vi "Shallow Copy.vi"(7 "Tree ID":string, 8 "Error In":errorcluster, 11 "Tree Manager":T1) -> (0 "Error Out":errorcluster, 3 "Tree Manager":T1, 5 "Unique ID of Copied Tree":string)   [LabVIEW 2016, in "Tree Manager.lvclass"]
doc: "Shallow copy of a Tree and its attributes. Does not copy the Children of the Tree. On all attributes that are Tree Data types a Copy method is invoked. Overwrite the Copy the method in child types of Tree Data to implement special copying mechanism. The Default mechanism is copying by values i.e. LV fork."
uses:
  Tree Manager.lvclass
  Typedefs/Session Handle.ctl
  Tree Manager.lvclass/Tree Manager.ctl
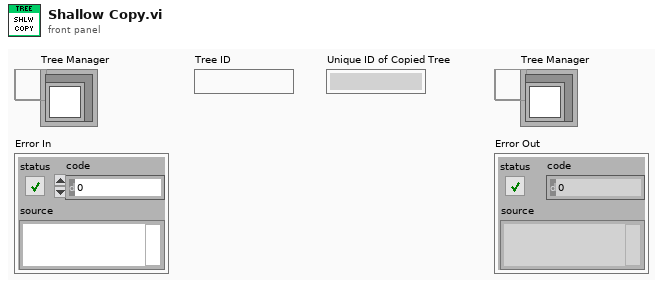
[diagram p1: front panel]
types:
  T1 = typedef "Tree Manager.lvclass/Session Handle.ctl" = refnum<data-value>
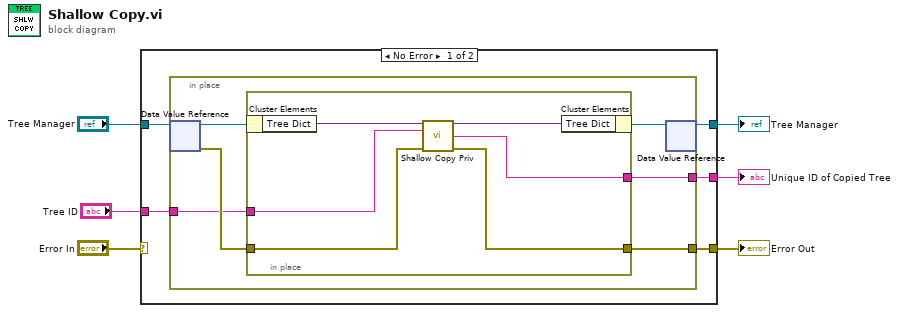
[diagram p0: block diagram]
diagram:
  n1 = case shown="No Error" "Error In" {
    selector: "Error In" -> [_ w24]
    tunnel: "Tree Manager" -> [w11 w25]
    tunnel: [w10 w25] -> w5
    tunnel: [w9 w24] -> w3
    tunnel: "Tree ID" -> [w8 _]
    tunnel: [w7 _] -> w1
    frame No Error {
      n2 = in-place {
        in-place-border: [w16] -> w9
        in-place-border: w8 -> [w13]
        in-place-border: [w12] -> w7
        n3 = in-place-dvr #1(w11) -> (w17:refnum<class "Tree Manager.lvclass">, w14:errorcluster)
        n4 = in-place {
          in-place-border: [w20] -> w16
          in-place-border: w14 -> [w21]
          in-place-border: w13 -> [w19]
          in-place-border: [w18] -> w12
          n5 = in-place-cluster #2(w17) -> ("Tree Dict"=w23:variant)
          n6 = call "Shallow Copy Priv.vi"("Tree Dictionary In"=w23, "Unique ID"=w19, "error in"=w21) -> ("Tree Dictionary Out"=w22:variant, "ID"=w18:string, "error out"=w20:errorcluster)  [unwired: 10 in]
          n7 = in-place-cluster #2("Tree Dict"=w22) -> (w15:refnum<class "Tree Manager.lvclass">)
        }
        n8 = in-place-dvr #1(w15) -> (w10:T1)  [unwired: 1 out]
      }
    }
    frame Error {
    }
  }
  "Tree Manager" <- w5
  "Error Out" <- w3
  "Unique ID of Copied Tree" <- w1
